vi "AVS_GetVersionInfo.vi"(0 "a_hDevice":i32, 7 "a_pFPGAVersion":i8[](array[numeric]), 9 "a_pFirmwareVersion":i8[](array[numeric]), 11 "a_pDLLVersion":i8[](array[numeric])) -> (4 "Output Value":i32, 8 "a_pFPGAVersion":i8[](array[numeric]), 10 "a_pFirmwareVersion":i8[](array[numeric]), 15 "a_pDLLVersion":i8[](array[numeric]))   [LabVIEW 2018]
uses:
  avaspecx64.dll
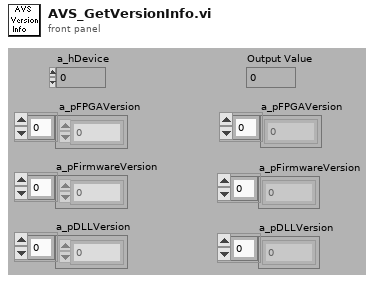
[diagram p1: front panel]
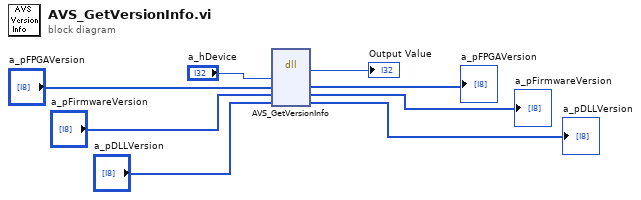
[diagram p0: block diagram]
diagram:
  n1 = dll-call lib="C:/AvaSpecX64-DLL_9.7/examples/LabView/LabViewSingleChan/avaspecx64.dll" fn="AVS_GetVersionInfo"("a_hDevice"="a_hDevice", "a_pFPGAVersion"="a_pFPGAVersion", "a_pFirmwareVersion"="a_pFirmwareVersion", "a_pDLLVersion"="a_pDLLVersion") -> ("return type"=→"Output Value":i32, "a_pFPGAVersion"=→"a_pFPGAVersion":i8[], "a_pFirmwareVersion"=→"a_pFirmwareVersion":i8[], "a_pDLLVersion"=→"a_pDLLVersion":i8[])  [unwired: 4 in, 2 out]
